vi "Bundle by name.vi"() -> ()   [LabVIEW 2015]
panel:
  in  "VI Refnum":refnum<vi>
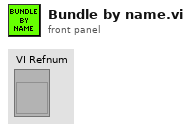
[diagram p1: front panel]
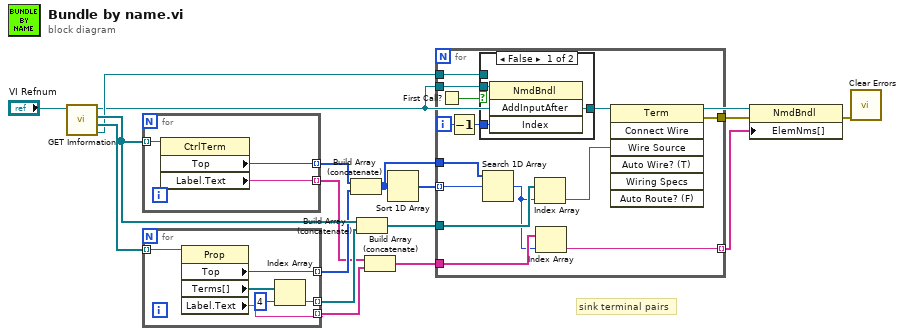
[diagram p0: block diagram]
diagram:
  # "sink terminal pairs"
  n1 = call "GET Imformation.vi"("VI Refnum"="VI Refnum") -> ("Term Refnum"=w8:refnum<vi>, "Property Reference"=w11:refnum<vi>[], "Terms Reference"=w15:refnum<vi>[], "Bundle Reference"=w5:refnum<vi>)  [unwired: 6 in, 1 out]
  n2 = for {
    tunnel: w15 -> [w20] mode=indexing
    tunnel: [w19] -> w16 mode=indexing
    tunnel: [w18] -> w4 mode=indexing
    n3 = property class="CtrlTerm"(reference=w20) -> ("Top"=w19:i32, "Label.Text"=w18:string)  [unwired: 1 in, 2 out]
  }
  n4 = for {
    tunnel: w11 -> [w24] mode=indexing
    tunnel: [w23] -> w10 mode=indexing
    tunnel: [w22] -> w9 mode=indexing
    tunnel: [w21] -> w3 mode=indexing
    n5 = property class="Prop"(reference=w24) -> ("Top"=w22:i32, "Terms[]"=w26:refnum<vi>[], "Label.Text"=w21:string)  [unwired: 1 in, 2 out]
    n6 = Index Array(array=w26, index=4) -> (element=w23:refnum<vi>)
  }
  n7 = Build Array (concatenate)(w16, w9) -> (w13:i32[])
  n8 = Build Array (concatenate)(w15, w10) -> (w14:refnum<vi>[])
  n9 = Build Array (concatenate)(w4, w3) -> (w2:string[])
  n10 = Sort 1D Array(array=w13) -> (sorted array=w12:i32[])
  n11 = for {
    tunnel: w12 -> [w38] mode=indexing
    tunnel: w14 -> [w40]
    tunnel: w13 -> [w39]
    tunnel: w8 -> [w35]
    tunnel: w5 -> [w34]
    tunnel: [w27] -> w7 mode=indexing
    tunnel: [w30] -> w6
    tunnel: w2 -> [w29]
    i -> [w33]
    n12 = First Call?() -> (First Call?: T/F=w37:bool)
    n13 = Decrement(x=w33) -> (x-1=w36:i32)
    n14 = case shown="False" w37 {
      tunnel: w34 -> [w43 _]
      tunnel: w36 -> [w42 _]
      tunnel: [w41 w44] -> w32
      tunnel: w35 -> [_ w44]
      frame False {
        n15 = invoke class="NmdBndl" method="AddInputAfter"(reference=w43, "Index"=w42) -> ("AddInputAfter"=w41:refnum<vi>)  [unwired: 2 in, 3 out]
      }
      frame True {
      }
    }
    n16 = Search 1D Array(1D array=w39, element=w38) -> (index of element=w28:i32)  [unwired: 1 in]
    n17 = Index Array(array=w40, index=w28) -> (element=w31:refnum<vi>)
    n18 = Index Array(array=w29, index=w28) -> (element=w27:string)
    n19 = invoke class="Term" method="Connect Wire"(reference=w32, "Wire Source"=w31) -> (error out=w30:errorcluster)  [unwired: 5 in, 6 out]
  }
  n20 = property class="NmdBndl"(reference=w5, error in=w6, "ElemNms[]"=w7) -> (error out=w1:errorcluster)  [unwired: 1 out]
  n21 = call <vilib>:"Clear Errors.vi"("error in (no error)"=w1) -> ()  [unwired: 5 in, 2 out]
